vi "ExecuteGrSimTestPasse.vi"(0 "RandomEnemyPoints":dbl[][](array[numeric]), 4 "Number of Points":i32, 5 "Atacando contra?":bool, 6 "Replace Robots":bool, 7 "IA State Input":T3, 8 "Região do campo\nTeste Passe":enum16{"3", "2", "1", "0", "-1", "-2", "-3"}(ring), 9 "reset":bool, 10 "id":i32, 11 "RandomAllyPoints":dbl[][](array[numeric])) -> (1 "kick num":i32, 2 "Replace active":bool, 3 "grSim replacement":cluster{"robots":T1[], "ball":T2}={"robots"=[{"x"=0.0, "y"=-450.0, "dir"=0.0, "yellowteam"=FALSE, "id"=0}, {"x"=0.0, "y"=-270.0, "dir"=0.0, "yellowteam"=FALSE, "id"=1}, {"x"=0.0, "y"=-90.0, "dir"=0.0, "yellowteam"=FALSE, "id"=2}, {"x"=0.0, "y"=90.0, "dir"=0.0, "yellowteam"=FALSE, "id"=3}, {"x"=0.0, "y"=270.0, "dir"=0.0, "yellowteam"=FALSE, "id"=4}, {"x"=0.0, "y"=450.0, "dir"=0.0, "yellowteam"=FALSE, "id"=5}], "ball"={"x"=0.0, "y"=0.0, "vx"=0.0, "vy"=0.0}})   [LabVIEW 2017]
uses:
  Core/AI Input.ctl
  Core/AI Robot.ctl
  Intel/Functions Enum.ctl
  Intel/AttackerStates.ctl
  Path Planning/RRT/PathDests.ctl
  Path Planning/RRT/PathDest.ctl
  Core/AI Ball.ctl
  Core/Field Size.ctl
  Core/AI Judge.ctl
  Intel/Command Enum.ctl
  Util/Events/Events.ctl
  grSim RobotReplacement.ctl
  grSim_BallReplacement.ctl
panel:
  in  "Time":enum16{"Azul", "Amarelo"}(ring) caption="Enum"
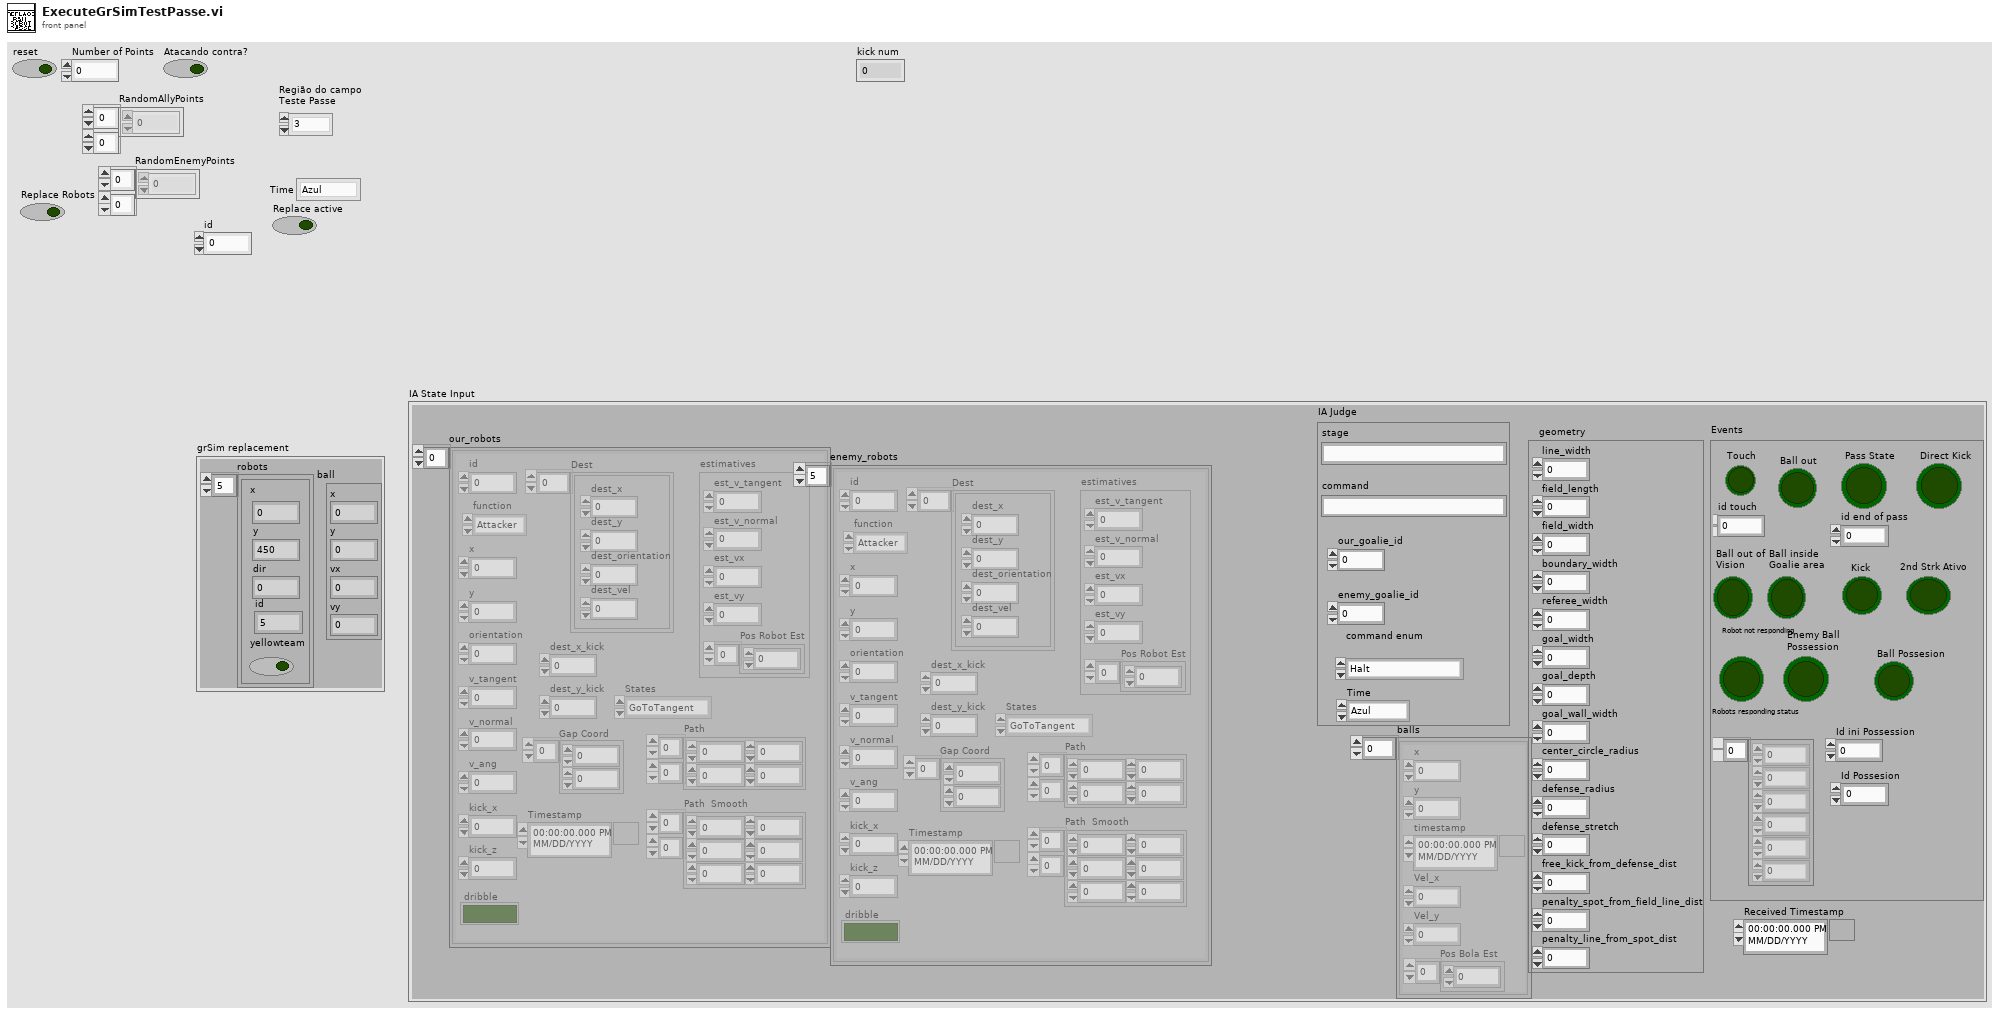
[diagram p1: front panel]
types:
  T1 = typedef "grSim RobotReplacement.ctl" = cluster{"x":dbl, "y":dbl, "dir":dbl, "yellowteam":bool, "id":u32}
  T2 = typedef "grSim_BallReplacement.ctl" = cluster{"x":dbl, "y":dbl, "vx":dbl, "vy":dbl}
  T3 = typedef "AI Input.ctl" = cluster{"our_robots":T4[], "enemy_robots":T4[], "balls":T9[], "geometry":T10, "IA Judge":T11, "Received Timestamp":timestamp, "Events":T13}
  T4 = typedef "AI Robot.ctl" = cluster{"id":u32, "function":T5, "x":dbl, "y":dbl, "orientation":dbl, "v_tangent":dbl, "v_normal":dbl, "v_ang":dbl, "kick_x":dbl, "kick_z":dbl, "dribble":bool, "Timestamp":timestamp, "estimatives":cluster{"est_v_tangent":dbl, "est_v_normal":dbl, "est_vx":dbl, "est_vy":dbl, "Pos Robot Est":dbl[]}, "dest_x_kick":dbl, "dest_y_kick":dbl, "Gap Coord":dbl[], "States":T6, "Path ":dbl[][], "Path  Smooth":dbl[][], "Dest":T7}
  T5 = typedef "Functions Enum.ctl" = enum16{"2nd Striker", "Attacker", "Goalie", "Defender", "Striker", "Goto 0", "Dummy", "Kicker", "ZigZag 0", "ZigZag 1", "ZigZag 2", "ZigZag 3", "ZigZag 4", "ZigZag 5", "ZigZag 6", "ZigZag 7", "ZigZag 8", ""}
  T6 = typedef "AttackerStates.ctl" = enum16{"Pass", "GoToTangent", "BallGetting", "GoToKick", ""}
  T7 = typedef "PathDests.ctl" = T8[]
  T8 = typedef "PathDest.ctl" = cluster{"dest_x":dbl, "dest_y":dbl, "dest_orientation":dbl, "dest_vel":dbl}
  T9 = typedef "AI Ball.ctl" = cluster{"x":dbl, "y":dbl, "timestamp":timestamp, "Vel_x":dbl, "Vel_y":dbl, "Pos Bola Est":dbl[]}
  T10 = typedef "Field Size.ctl" = cluster{"line_width":u32, "field_length":u32, "field_width":u32, "boundary_width":u32, "referee_width":u32, "goal_width":u32, "goal_depth":u32, "goal_wall_width":u32, "center_circle_radius":u32, "defense_radius":u32, "defense_stretch":u32, "free_kick_from_defense_dist":u32, "penalty_spot_from_field_line_dist":u32, "penalty_line_from_spot_dist":u32}
  T11 = typedef "AI Judge.ctl" = cluster{"stage":string, "command":string, "our_goalie_id":dbl, "enemy_goalie_id":dbl, "command enum":T12, "Time":enum16{"Azul", "Amarelo"}}
  T12 = typedef "Command Enum.ctl" = enum16{"Halt", "Stop", "Force Start", "PKA Normal Start", "Prepare Kickoff Ally", "PKE Normal Start", "Prepare Kickoff Enemy", "Prepare Penalty Ally", "PPA Normal Start", "Prepare Penalty Enemy", "PPE Normal Start", "Direct Free Enemy", "Direct Free Ally", "Indirect Free Enemy", "Indirect Free Ally", "Timeout Enemy", "Timeout Ally", "Goal Enemy", "Goal Ally", "Ball Placement Enemy", "Ball Placement Ally", "Normal Half Time", "Extra Time Break", "Extra Half Time", "None", "Post Game"}
  T13 = typedef "Events.ctl" = cluster{"Touch":bool, "Ball out":bool, "id touch":dbl, "Ball out of \nVision":bool, "Ball inside \nGoalie area":bool, "Robot not responding":bool, "Robots responding status":dbl[], "Enemy Ball \nPossession":bool, "Pass State":bool, "id end of pass":dbl, "Kick":bool, "Id ini Possession":dbl, "Ball Possesion":bool, "Id Possesion":dbl, "Direct Kick":bool, "2nd Strk Ativo":bool}
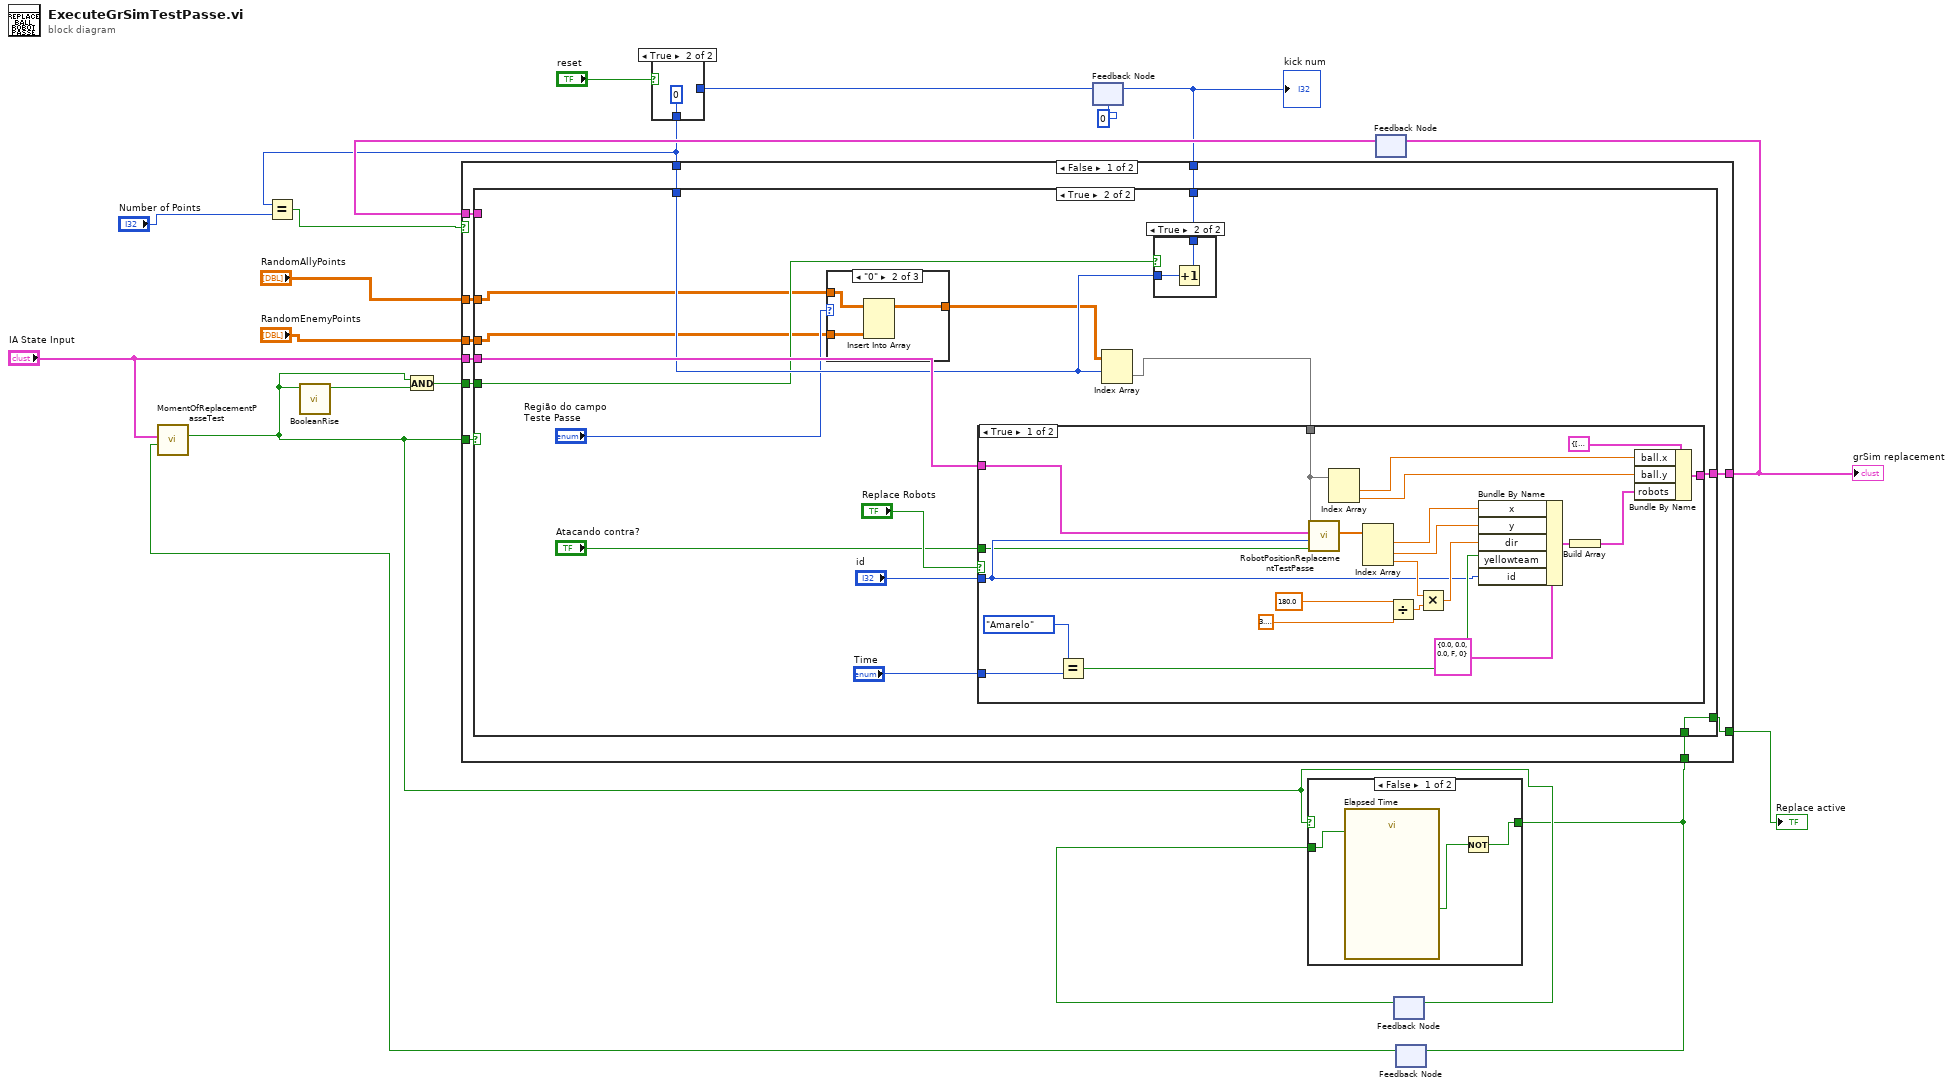
[diagram p0: block diagram]
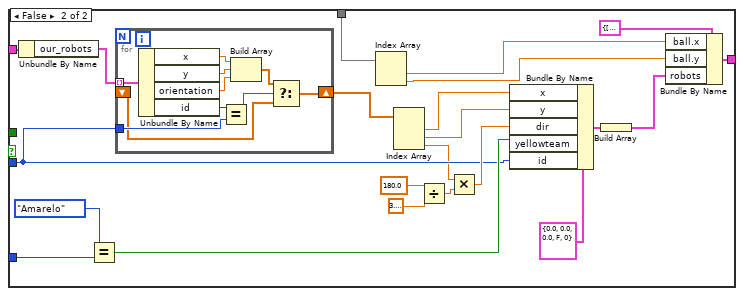
[diagram p6: hidden frame]
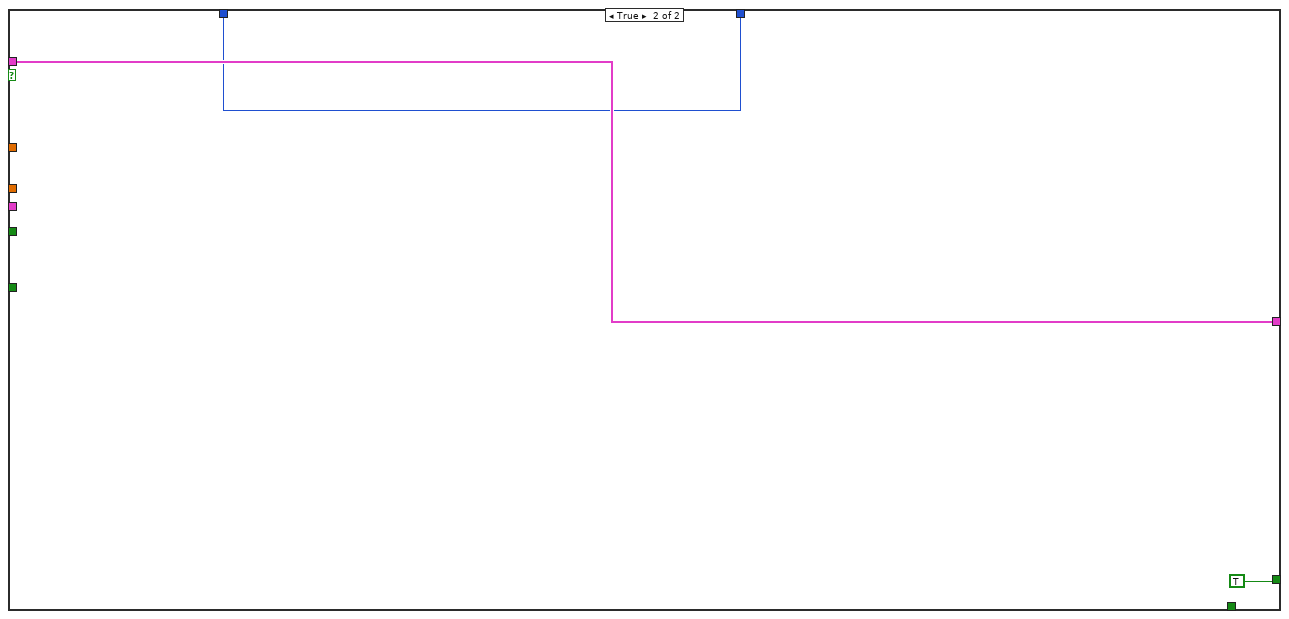
[diagram p7: hidden frame]
diagram:
  n1 = feedback #1(0) -> (w9:i32)
  n2 = case shown="True" "reset" {
    tunnel: w9 -> [w20 _]
    tunnel: [w20 0] -> w6
    frame False {
    }
    frame True {
    }
  }
  n3 = Equal?(x=w6, y="Number of Points") -> (x = y?=w5:bool)
  n4 = feedback #2() -> (w19:cluster{"robots":T1[], "ball":T2})  [unwired: 1 in]
  n5 = feedback #3() -> (w18:bool)  [unwired: 1 in]
  n6 = feedback #4() -> (w15:bool)  [unwired: 1 in]
  n7 = call "MomentOfReplacementPasseTest.vi"("Replace active"=w15, "IA State Input"="IA State Input") -> ("Time to replace?"=w10:bool)  [unwired: 9 in]
  n8 = call "BooleanRise.vi"("Test Mode On"=w10) -> ("Boolean"=w11:bool)  [unwired: 10 in]
  n9 = And(x=w10, y=w11) -> (x .and. y?=w12:bool)
  n10 = case shown="False" w10 {
    selector: w10 -> [_ w25]
    tunnel: [w24 w25] -> w4
    tunnel: w18 -> [w22 _]
    frame False {
      n11 = call "Elapsed Time"("Reset"=w22) -> ("Time has Elapsed"=w23:bool)  [unwired: 11 in, 7 out]
      n12 = Not(x=w23) -> (.not. x?=w24:bool)
    }
    frame True {
    }
  }
  n13 = case shown="False" w5 {
    tunnel: w19 -> [w36 w118]
    tunnel: [w35 w118] -> w17
    tunnel: "IA State Input" -> [w34 _]
    tunnel: "RandomAllyPoints" -> [w33 _]
    tunnel: [w32 w117] -> w13
    tunnel: w12 -> [w31 _]
    tunnel: w10 -> [w30 _]
    tunnel: w6 -> [w29 w117]
    tunnel: w4 -> [w27 _]
    tunnel: [w28 TRUE] -> w3
    tunnel: "RandomEnemyPoints" -> [w26 _]
    frame False {
      n14 = case shown="True" w30 {
        tunnel: [w39 w54] -> w35
        tunnel: w34 -> [_ w51]
        tunnel: w36 -> [w39 _]
        tunnel: w33 -> [_ w42]
        tunnel: w29 -> [w38 w48]
        tunnel: [w38 w47] -> w32
        tunnel: w31 -> [_ w46]
        tunnel: [w37 w45] -> w28
        tunnel: w27 -> [w37 w45]
        tunnel: w26 -> [_ w41]
        frame False {
        }
        frame True {
          n15 = case shown="\"0\"" "Região do campo\nTeste Passe" {
            tunnel: w42 -> [w55 w58 _]
            tunnel: w41 -> [_ w57 w59]
            tunnel: [w55 w56 w59] -> w40
            frame "-1".."-3" {
            }
            frame "0" {
              n16 = Insert Into Array(array=w58, new element=w57) -> (w56:dbl[][])  [unwired: 2 in]
            }
            frame "3".."1" {
            }
          }
          n17 = Index Array(array=w40, index (row)=w48) -> (element=w53:dbl[])  [unwired: 1 in]
          n18 = case shown="True" "Replace Robots" {
            tunnel: [w84 w106] -> w54
            tunnel: w53 -> [w67 w88]
            tunnel: "Time" -> [w80 w102]
            tunnel: w51 -> [w75 w95]
            tunnel: "id" -> [w68 w93]
            tunnel: "Atacando contra?" -> [w63 _]
            frame True {
              n19 = Equal?(x=enum16{"Azul", "Amarelo"}."Amarelo", y=w80) -> (x = y?=w78:bool)
              n20 = call "RobotPositionReplacementTestPasse.vi"("Atacando contra?"=w63, "id"=w68, "IA State Input"=w75, "Position Ball"=w67) -> ("Position Robot"=w77:dbl[])  [unwired: 5 in]
              n21 = Index Array(array=w67) -> (element #1=w66:dbl, element #2=w65:dbl)  [unwired: 2 in]
              n22 = Index Array(array=w77) -> (element #1=w76:dbl, element #2=w74:dbl, element #3=w69:dbl)  [unwired: 3 in]
              n23 = Divide(x=180.0, y=3.141592653589793) -> (x/y=w72:dbl)
              n24 = Multiply(x=w69, y=w72) -> (x*y=w73:dbl)
              n25 = Bundle By Name(cluster=T1 {"x"=0.0, "y"=0.0, "dir"=0.0, "yellowteam"=FALSE, "id"=0} ("element"), "x"=w76, "y"=w74, "dir"=w73, "yellowteam"=w78, "id"=w68) -> (w82:T1)
              n26 = Build Array(w82) -> (w81:T1[])
              n27 = Bundle By Name(cluster=cluster{"robots":T1[], "ball":T2} {"robots"=[{"x"=0.0, "y"=-450.0, "dir"=0.0, "yellowteam"=FALSE, "id"=0}, {"x"=0.0, "y"=-270.0, "dir"=0.0, "yellowteam"=FALSE, "id"=1}, {"x"=0.0, "y"=-90.0, "dir"=0.0, "yellowteam"=FALSE, "id"=2}, {"x"=0.0, "y"=90.0, "dir"=0.0, "yellowteam"=FALSE, "id"=3}, {"x"=0.0, "y"=270.0, "dir"=0.0, "yellowteam"=FALSE, "id"=4}, {"x"=0.0, "y"=450.0, "dir"=0.0, "yellowteam"=FALSE, "id"=5}], "ball"={"x"=0.0, "y"=0.0, "vx"=0.0, "vy"=0.0}} ("grSim replacement"), "ball.x"=w66, "ball.y"=w65, "robots"=w81) -> (w84:cluster{"robots":T1[], "ball":T2})
            }
            frame False {
              n28 = Unbundle By Name(w95) -> ("our_robots"=w94:T4[])
              n29 = Equal?(x=enum16{"Azul", "Amarelo"}."Amarelo", y=w102) -> (x = y?=w100:bool)
              n30 = for {
                tunnel: w94 -> [w116] mode=indexing
                tunnel: w93 -> [w114]
                shift-right: [w108] -> w92
                shift-left: _ -> [w107]
                n31 = Unbundle By Name(w116) -> ("x"=w113:dbl, "y"=w112:dbl, "orientation"=w111:dbl, "id"=w115:u32)
                n32 = Equal?(x=w115, y=w114) -> (x = y?=w110:bool)
                n33 = Build Array(w113, w112, w111) -> (w109:dbl[])
                n34 = Select(t=w109, s=w110, f=w107) -> (s? t:f=w108:dbl[])
              }
              n35 = Index Array(array=w88) -> (element #1=w87:dbl, element #2=w86:dbl)  [unwired: 2 in]
              n36 = Index Array(array=w92) -> (element #1=w91:dbl, element #2=w89:dbl, element #3=w90:dbl)  [unwired: 3 in]
              n37 = Divide(x=180.0, y=3.141592653589793) -> (x/y=w98:dbl)
              n38 = Multiply(x=w90, y=w98) -> (x*y=w99:dbl)
              n39 = Bundle By Name(cluster=T1 {"x"=0.0, "y"=0.0, "dir"=0.0, "yellowteam"=FALSE, "id"=0} ("element"), "x"=w91, "y"=w89, "dir"=w99, "yellowteam"=w100, "id"=w93) -> (w104:T1)
              n40 = Build Array(w104) -> (w103:T1[])
              n41 = Bundle By Name(cluster=cluster{"robots":T1[], "ball":T2} {"robots"=[{"x"=0.0, "y"=-450.0, "dir"=0.0, "yellowteam"=FALSE, "id"=0}, {"x"=0.0, "y"=-270.0, "dir"=0.0, "yellowteam"=FALSE, "id"=1}, {"x"=0.0, "y"=-90.0, "dir"=0.0, "yellowteam"=FALSE, "id"=2}, {"x"=0.0, "y"=90.0, "dir"=0.0, "yellowteam"=FALSE, "id"=3}, {"x"=0.0, "y"=270.0, "dir"=0.0, "yellowteam"=FALSE, "id"=4}, {"x"=0.0, "y"=450.0, "dir"=0.0, "yellowteam"=FALSE, "id"=5}], "ball"={"x"=0.0, "y"=0.0, "vx"=0.0, "vy"=0.0}} ("grSim replacement"), "ball.x"=w87, "ball.y"=w86, "robots"=w103) -> (w106:cluster{"robots":T1[], "ball":T2})
            }
          }
          n42 = case shown="True" w46 {
            tunnel: w48 -> [w60 w62]
            tunnel: [w60 w61] -> w47
            frame False {
            }
            frame True {
              n43 = Increment(x=w62) -> (x+1=w61:i32)
            }
          }
        }
      }
    }
    frame True {
    }
  }
  "grSim replacement" <- w17
  "Replace active" <- w3
  "kick num" <- w13
  n44 = feedback-in #1(w13) -> ()
  n45 = feedback-in #2(w17) -> ()
  n46 = feedback-in #3(w10) -> ()
  n47 = feedback-in #4(w4) -> ()
